vi "denomination.vi"() -> ()   [LabVIEW 2019]
panel:
  out "Denominations":i32[][](array[numeric])
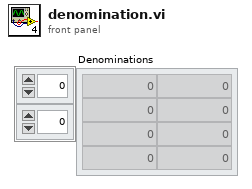
[diagram p1: front panel]
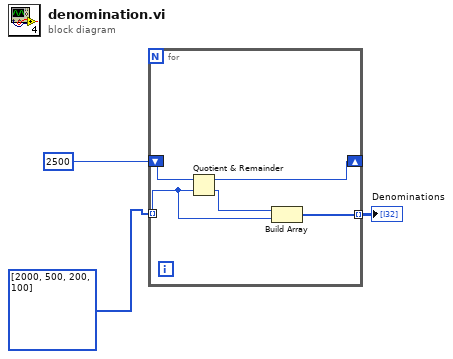
[diagram p0: block diagram]
diagram:
  n1 = for {
    tunnel: i32[] [2000, 500, 200, 100] -> [w7] mode=indexing
    shift-right: [w5] -> _
    shift-left: 2500 -> [w8]
    tunnel: [w6] -> w1 mode=indexing
    n2 = Quotient & Remainder(x=w8, y=w7) -> (x-y*floor(x/y)=w5:i32, floor(x/y)=w4:i32)
    n3 = Build Array(w4, w7) -> (w6:i32[])
  }
  "Denominations" <- w1
